vi "Register gRPC Methods.vi"(8 "error in (no error)":errorcluster, 11 "Template Server in":refnum<class "RouteGuide.lvclass">) -> (0 "error out":errorcluster, 3 "Template Server out":refnum<class "RouteGuide.lvclass">)   [LabVIEW 2019, in "Generated_server.lvlib" / "RouteGuide.lvclass"]
uses:
  RouteGuide.lvclass
  typeDefs/Server Internal UEs.ctl
  typeDefs/Server Internal Message.ctl
  typeDefs/Server gRPC UEs.ctl
  <vilib>/gRPC/LabVIEW gRPC Library/Server API/typeDefs/gRPCId Cluster.ctl
  <vilib>/gRPC/LabVIEW gRPC Library/Shared/grpcId.ctl
  RouteGuide.lvclass/RouteGuide.ctl
  <vilib>/gRPC/LabVIEW gRPC Library/grpc-lvsupport-release.lvlib
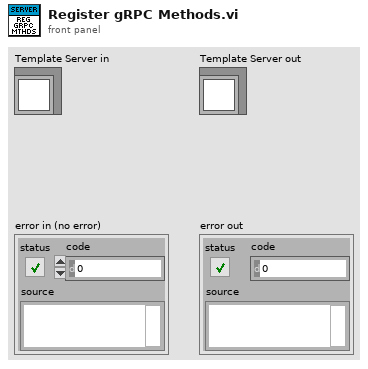
[diagram p1: front panel]
types:
  T1 = typedef "Generated_server.lvlib/RouteGuide.lvclass/Server gRPC UEs.ctl" = cluster{"RouteGuide UnaryMethod gRPC UE":refnum<user-event>, "RouteGuide ServerStreamingMethod gRPC UE":refnum<user-event>, "RouteGuide ClientStreamingMethod gRPC UE":refnum<user-event>, "RouteGuide BidirectionalStreamingMethod gRPC UE":refnum<user-event>}
  T2 = typedef "Generated_server.lvlib/RouteGuide.lvclass/Server Internal UEs.ctl" = cluster{"RouteGuide UnaryMethod Internal UE":refnum<user-event>, "RouteGuide ServerStreamingMethod Internal UE":refnum<user-event>, "RouteGuide ClientStreamingMethod Internal UE":refnum<user-event>, "RouteGuide BidirectionalStreamingMethod Internal UE":refnum<user-event>}
  T3 = typedef "grpc-lvsupport-release.lvlib/grpcId.ctl" = u64
  T4 = typedef "Generated_server.lvlib/RouteGuide.lvclass/Server Internal Message UE.ctl" = refnum<user-event>
  T5 = typedef "grpc-lvsupport-release.lvlib/gRPCId Cluster UE.ctl" = refnum<user-event>
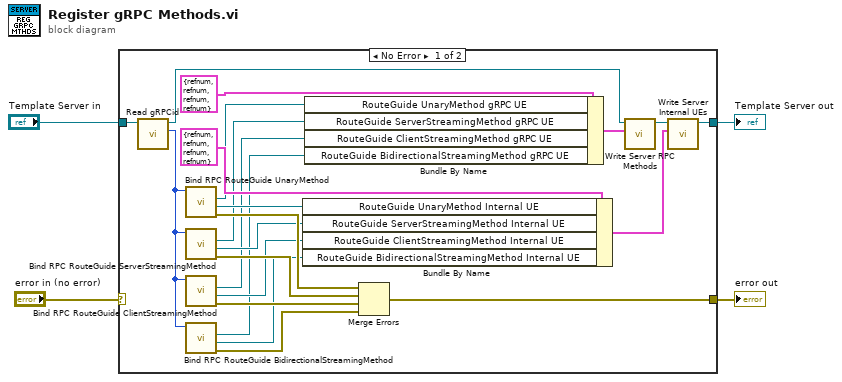
[diagram p0: block diagram]
diagram:
  n1 = case shown="No Error" "error in (no error)" {
    selector: "error in (no error)" -> [_ w27]
    tunnel: "Template Server in" -> [w18 w28]
    tunnel: [w26 w27] -> w3
    tunnel: [w25 w28] -> w2
    frame No Error {
      n2 = call-dynamic "Read gRPCid.vi"("iService in"=w18) -> ("gRPCid"=w17:T3, "iService out"=w19:refnum<class "RouteGuide.lvclass">)  [unwired: 8 in, 1 out]
      n3 = call "Bind RPC RouteGuide UnaryMethod.vi"("gRPCid server in"=w17) -> ("error out"=w16:errorcluster, "RouteGuide UnaryMethod Internal UE"=w14:T4, "RouteGuide UnaryMethod gRPC UE"=w15:T5)  [unwired: 7 in, 1 out]
      n4 = call "Bind RPC RouteGuide ServerStreamingMethod.vi"("gRPCid server in"=w17) -> ("error out"=w13:errorcluster, "RouteGuide ServerStreamingMethod Internal UE"=w11:T4, "RouteGuide ServerStreamingMethod gRPC UE"=w12:T5)  [unwired: 7 in, 1 out]
      n5 = call "Bind RPC RouteGuide ClientStreamingMethod.vi"("gRPCid server in"=w17) -> ("error out"=w10:errorcluster, "RouteGuide ClientStreamingMethod Internal UE"=w8:T4, "RouteGuide ClientStreamingMethod gRPC UE"=w9:T5)  [unwired: 7 in, 1 out]
      n6 = call "Bind RPC RouteGuide BidirectionalStreamingMethod.vi"("gRPCid server in"=w17) -> ("error out"=w7:errorcluster, "RouteGuide BidirectionalStreamingMethod Internal UE"=w5:T4, "RouteGuide BidirectionalStreamingMethod gRPC UE"=w6:T5)  [unwired: 7 in, 1 out]
      n7 = Bundle By Name ("Bundle Internal UEs")(cluster=T2 {"RouteGuide UnaryMethod Internal UE"=refnum, "RouteGuide ServerStreamingMethod Internal UE"=refnum, "RouteGuide ClientStreamingMethod Internal UE"=refnum, "RouteGuide BidirectionalStreamingMethod Internal UE"=refnum} ("Server Internal UEs"), "RouteGuide UnaryMethod Internal UE"=w14, "RouteGuide ServerStreamingMethod Internal UE"=w11, "RouteGuide ClientStreamingMethod Internal UE"=w8, "RouteGuide BidirectionalStreamingMethod Internal UE"=w5) -> (w24:T2)
      n8 = Bundle By Name ("Bundle gRPC UEs")(cluster=T1 {"RouteGuide UnaryMethod gRPC UE"=refnum, "RouteGuide ServerStreamingMethod gRPC UE"=refnum, "RouteGuide ClientStreamingMethod gRPC UE"=refnum, "RouteGuide BidirectionalStreamingMethod gRPC UE"=refnum} ("gRPC Server Method Events"), "RouteGuide UnaryMethod gRPC UE"=w15, "RouteGuide ServerStreamingMethod gRPC UE"=w12, "RouteGuide ClientStreamingMethod gRPC UE"=w9, "RouteGuide BidirectionalStreamingMethod gRPC UE"=w6) -> (w21:T1)
      n9 = Merge Errors(w16, w13, w10, w7) -> (w26:errorcluster)
      n10 = call "Write Server RPC Methods.vi"("Server RPC Methods"=w21, "SignalGeneratorService in"=w19) -> ("SignalGeneratorService out"=w22:refnum<class "RouteGuide.lvclass">)  [unwired: 8 in, 1 out]
      n11 = call "Write Server Internal UEs.vi"("Server Internal UEs"=w24, "SignalGeneratorService in"=w22) -> ("SignalGeneratorService out"=w25:refnum<class "RouteGuide.lvclass">)  [unwired: 8 in, 1 out]
    }
    frame Error {
    }
  }
  "error out" <- w3
  "Template Server out" <- w2
